vi "destroy semaphores.vi"(8 "error in (no error)":errorcluster, 11 "semaphores in":T1[](array[typedef])) -> (0 "error out":errorcluster)   [LabVIEW 2013, in "Shared Memory runtime.lvclass"]
uses:
  Shared Memory runtime.lvclass
  controls/semaphore data.ctl
  <vilib>/NI/Pthreads for LabVIEW on Linux RT/Classes/Semaphore/Controls/reference.ctl
  <vilib>/NI/Pthreads for LabVIEW on Linux RT/Classes/Semaphore/Semaphore.lvclass
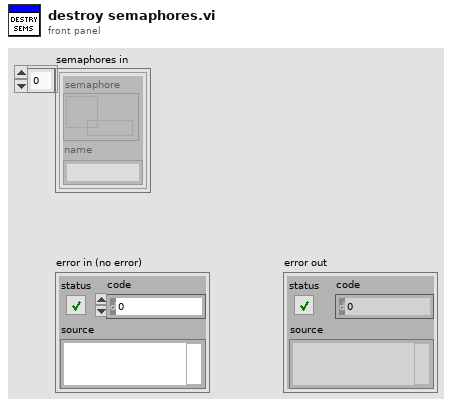
[diagram p1: front panel]
types:
  T1 = typedef "Shared Memory runtime.lvclass/semaphore data.ctl" = cluster{"semaphore":T2, "name":string}
  T2 = typedef "POSIX Threads.lvlib/Semaphore.lvclass/reference.ctl" = refnum<data-value>
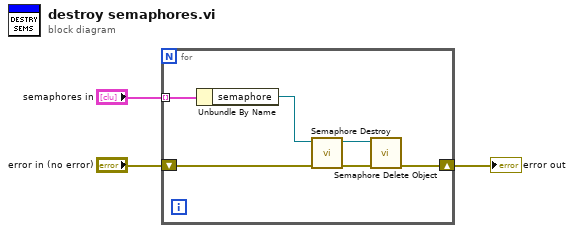
[diagram p0: block diagram]
diagram:
  n1 = for {
    tunnel: "semaphores in" -> [w6] mode=indexing
    shift-right: [w4] -> w1
    shift-left: "error in (no error)" -> [w7]
    n2 = Unbundle By Name(w6) -> ("semaphore"=w5:T2)
    n3 = call <vilib>:"Semaphore Destroy.vi"("error in (no error)"=w7, "Semaphore in"=w5) -> ("error out"=w8:errorcluster, "Semaphore out"=w9:T2)  [unwired: 8 in]
    n4 = call <vilib>:"Semaphore Delete Object.vi"("error in (no error)"=w8, "Semaphore in"=w9) -> ("error out"=w4:errorcluster)  [unwired: 8 in, 1 out]
  }
  "error out" <- w1
